vi "skil3.vi"() -> ()   [LabVIEW 2010]
uses:
  <vilib>/Utility/miscctls.llb/LVRectTypeDef.ctl
  lib/Global 2.vi
  <vilib>/Platform/browser.llb/Open URL in Default Browser (path).vi
panel:
  in  "Ed":bool
  in  "fv":bool
  in  "tm":bool
  out "mode":bool caption="Расписание"
  out "Table":string[][](table)
  out "User":string
  out "Device:Temperature":dbl format="%#4.0f"
  out "GPS:Status":i32(ring) items=["Uninitialized", "Antenna Error", "No Useable Satellites", "One Useable Satellite", "Two Useable Satellites", "Three Useable Satellites", "No GPS Time", "PDOP Too High", "Unuseable Satellite", "Fix Rejected", "Self Survey Complete", "Self Survey Not Complete"]
  out "d_h_m_s":dbl caption="в работе (дни, часы, минуты, секунды)" format="%<%D:%H:%M:%S>t"
  out "# elements in queue":i32 caption="Импульсов"
  in  "indexhtm":bool
  in  "stop 2":bool
  out "Get":bool caption="Датчики"
  out "Save2disk":bool caption="Диск"
  out "Files":i32 caption="Необработано"
  out "Send":bool caption="Сервер"
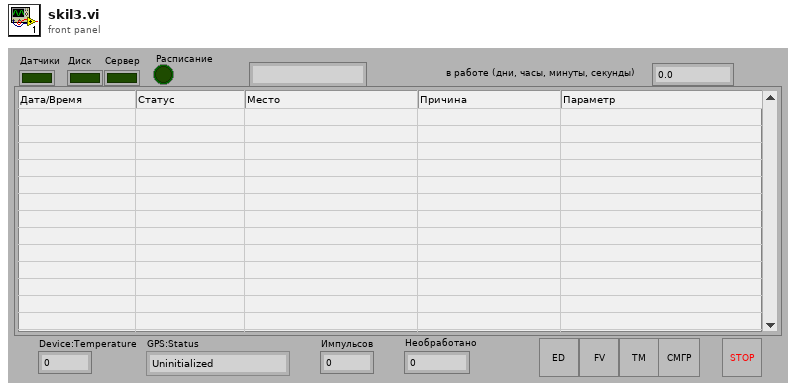
[diagram p1: front panel]
types:
  T1 = cluster{"seconds since 1Jan1904":timestamp, "error out":errorcluster}
  T2 = typedef "LVRectTypeDef.ctl" = cluster{"Left":i16, "Top":i16, "Right":i16, "Bottom":i16}
  T3 = cluster{cluster{"actualSamples":i32, "absoluteInitialX":dbl, "relativeInitialX":dbl, "xIncrement":dbl, "offset":dbl, "gain":dbl, "reserved1":dbl, "reserved2":dbl}[], "wfm":i16[][]}
  T4 = cluster{"adc handle":refnum<k15>, "PN":string, "KR":string}
  T5 = cluster{"seconds since 1Jan1904":timestamp, "error out":errorcluster}[]
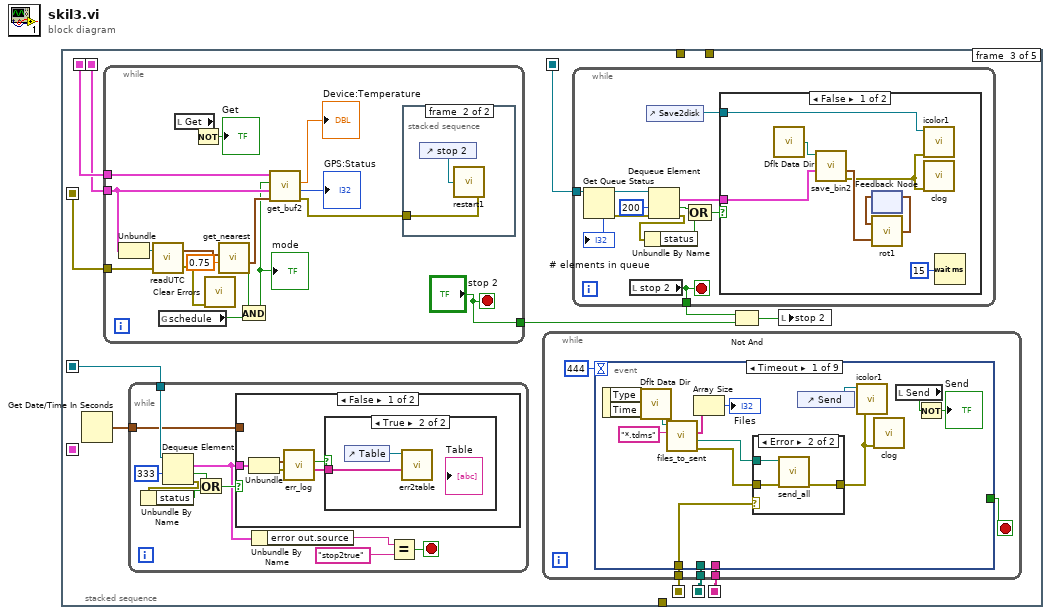
[diagram p0: block diagram]
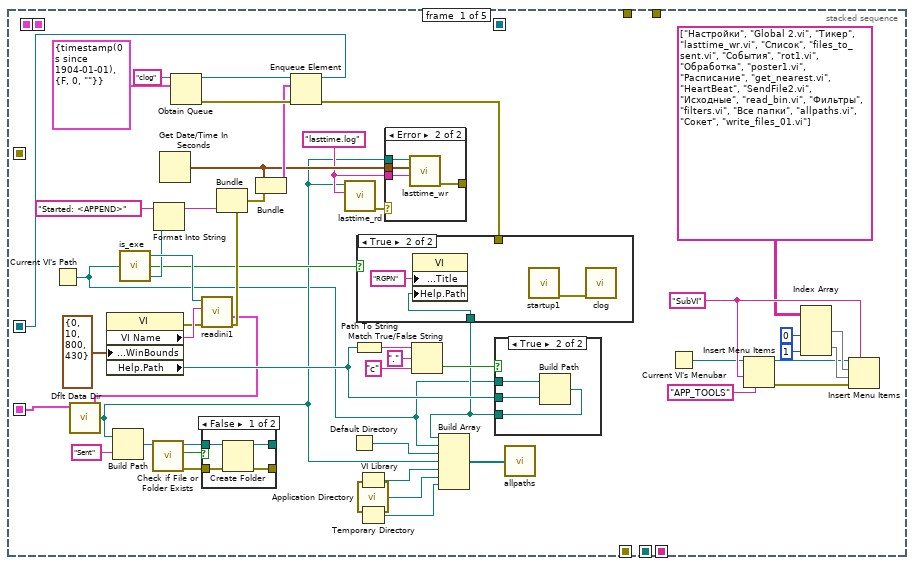
[diagram p2: hidden frame]
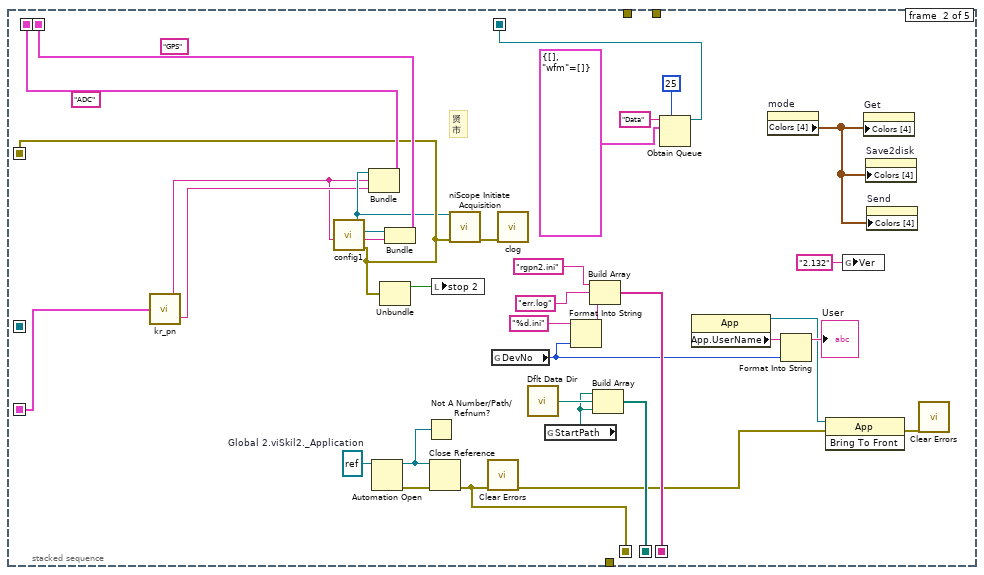
[diagram p7: hidden frame]
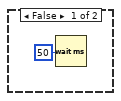
[diagram p8: hidden frame]
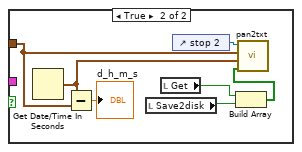
[diagram p9: hidden frame]
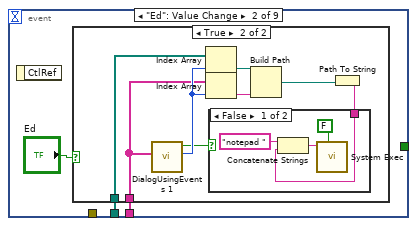
[diagram p11: hidden frame]
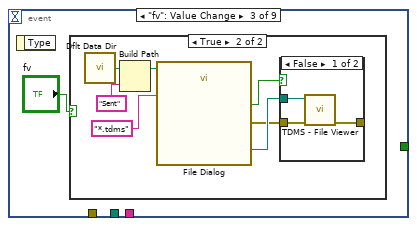
[diagram p14: hidden frame]
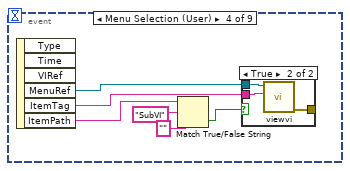
[diagram p17: hidden frame]
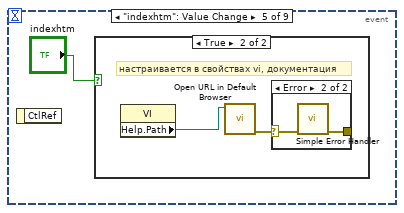
[diagram p19: hidden frame]
diagram:
  n1 = stacked-sequence {
    seq-local: [_ w93 _ _ _] -> [_ _ w113 w269 _]
    seq-local: [_ w101 _ _ _] -> [_ _ w112 w275 _]
    seq-local: [_ w97 _ _ _] -> [_ _ w110 w264 _]
    seq-local: [_ w98 _ _ _] -> [_ _ w111 w266 _]
    seq-local: [w20 _ _ _ _] -> [_ _ w109 w260 _]
    seq-local: [_ w84 _ _ _] -> [_ _ w108 _ _]
    seq-local: [_ w83 _ _ _] -> [_ _ w107 _ _]
    seq-local: [_ w74 _ _ _] -> [_ _ w102 _ _]
    seq-local: [w1 _ _ _ _] -> [_ w69 _ _ _]
    tunnel: [_ _ _ w256 _] -> _
    tunnel: [_ _ _ w255 _] -> _
    tunnel: [_ _ _ w252 _] -> _
    frame #0 {
      w6 = "lasttime.log" ("name or relative path")
      w40 = "SubVI"
      n2 = Current VI's Path() -> (path=w3:path)
      n3 = call <vilib>:"Dflt Data Dir.vi"() -> ("App:Default Data Directory"=w4:path)
      n4 = property class="VI"("Front Panel.WinBounds"=T2 {"Left"=0, "Top"=10, "Right"=800, "Bottom"=430} ("Front Panel Window:Window Bounds")) -> (error out=w47:errorcluster, "VI Name"=w49:string, "Help.Path"=w13:path)  [unwired: 2 in, 1 out]
      n5 = Build Path(base path=w4, name or relative path="Sent") -> (appended path=w44:path)
      n6 = call "is_exe.vi"("path"=w3) -> ("actual path"=w21:path, "exe?"=w19:bool, "ini path"=w48:path)  [unwired: 2 in]
      n7 = call <vilib>:"Check if File or Folder Exists.vi"("path"=w44) -> ("error out"=w41:errorcluster, "file or folder exists?"=w43:bool, "dup path"=w42:path)  [unwired: 8 in]
      n8 = Format Into String(initial string="Started: <APPEND>" ("string"), w21) -> (resulting string=w24:string)  [unwired: 2 in, 1 out]
      n9 = Get Date/Time In Seconds() -> (seconds since 1Jan1904=w7:timestamp)
      n10 = Obtain Queue(name (unnamed)="clog", element data type=T1 {"seconds since 1Jan1904"=timestamp(0 s since 1904-01-01), "error out"={"status"=FALSE, "code"=0, "source"=""}} ("output cluster")) -> (queue out=w28:refnum<queue>, error out=w27:errorcluster)  [unwired: 3 in, 1 out]
      n11 = call "readini1.vi"("error in (no error)"=w47, "section"=w49, "configuration file path"=w48) -> ("error out"=w26:errorcluster, "Dev_Gr"=w1:cluster{"DevNo":i32, "Group":string}[])  [unwired: 1 in, 2 out]
      n12 = case shown="False" w43 {
        tunnel: w42 -> [w64 w66]
        tunnel: w41 -> [w63 w65]
        tunnel: [w62 w66] -> _
        tunnel: [w61 w65] -> _
        frame False {
          n13 = Create Folder(path (use dialog)=w64, error in=w63) -> (created path=w62:path, error out=w61:errorcluster)  [unwired: 1 in, 1 out]
        }
        frame True {
        }
      }
      n14 = Bundle(cluster=w26, "source"=w24) -> (w23:errorcluster)  [unwired: 2 in]
      n15 = Bundle("seconds since 1Jan1904"=w7, "error out"=w23) -> (w22:T1)  [unwired: 1 in]
      n16 = Enqueue Element(queue=w28, element=w22, error in (no error)=w27) -> (queue out=w20:refnum<queue>, error out=w18:errorcluster)  [unwired: 1 in, 1 out]
      n17 = call "lasttime_rd.vi"("name or relative path"=w6, "base path"=w4) -> ("error out"=w5:errorcluster)  [unwired: 3 in, 2 out]
      n18 = Default Directory() -> (w15:path)
      n19 = Path To String(path=w13) -> (string=w12:string)
      n20 = VI Library() -> (path=w16:path)
      n21 = call <vilib>:"Application Directory.vi"() -> ("Application Directory"=w2:path)
      n22 = Temporary Directory() -> (w17:path)
      n23 = case shown="Error" w5 {
        tunnel: w7 -> [_ w53]
        tunnel: w6 -> [_ w52]
        tunnel: w4 -> [_ w51]
        tunnel: [_ w50] -> _
        frame No Error {
        }
        frame Error {
          n24 = call "lasttime_wr.vi"("name"=w52, "time stamp"=w53, "start Path"=w51) -> ("error out"=w50:errorcluster)  [unwired: 3 in, 1 out]
        }
      }
      n25 = Match True/False String(2:"c" ("false string"), 3:"." ("true string"), 4:w12) -> (0:w9:bool)  [unwired: 1 out]
      n26 = case shown="True" w9 {
        tunnel: w13 -> [w54 w57]
        tunnel: [w54 w56] -> w8
        tunnel: w3 -> [_ w55]
        frame False {
        }
        frame True {
          n27 = Build Path(base path=w55, name or relative path=w57) -> (appended path=w56:path)
        }
      }
      n28 = case shown="True" w19 {
        tunnel: w18 -> [_ _]
        tunnel: w8 -> [_ w58]
        frame False {
        }
        frame True {
          n29 = property class="VI"("Front Panel.Title"="RGPN" ("Front Panel Window:Title"), "Help.Path"=w58) -> ()  [unwired: 2 in, 2 out]
          n30 = call "startup1.vi"() -> ("error out"=w59:errorcluster)  [unwired: 7 in]
          n31 = call "clog.vi"("error"=w59) -> ()  [unwired: 7 in]
        }
      }
      n32 = Build Array(w8, w3, w15, w4, w16, w2, w17) -> (w14:path[])
      n33 = call "allpaths.vi"("Array"=w14) -> ()
      n34 = Current VI's Menubar() -> (w31:refnum<k9>)
      n35 = Insert Menu Items(4:"APP_TOOLS" ("after item"), 7:w40, 9:w31) -> (0:w33:errorcluster, 3:w32:refnum<k9>)  [unwired: 3 in, 1 out]
      n36 = Index Array(array=string[][] [["Настройки", "Global 2.vi"], ["Тикер", "lasttime_wr.vi"], ["Список", "files_to_sent.vi"], ["События", "rot1.vi"], ["Обработка", "poster1.vi"], ["Расписание", "get_nearest.vi"], ["HeartBeat", "SendFile2.vi"], ["Исходные", "read_bin.vi"], ["Фильтры", "filters.vi"], ["Все папки", "allpaths.vi"], ["Сокет", "write_files_01.vi"]], index (col) #1=0 ("disabled index (col)"), index (col) #2=1 ("index (col)")) -> (element #1=w36:string[], element #2=w37:string[])  [unwired: 2 in]
      n37 = Insert Menu Items(5:w40, 6:w33, 7:w37, 8:w36, 9:w32) -> ()  [unwired: 1 in, 3 out]
    }
    frame #1 {
      w75 = refnum<k7> refnum  # Global 2.viSkil2._Application
      (unwired) "GPS"
      (unwired) "ADC"
      # "贤\n市"
      n38 = call "kr_pn.vi"("Dev_Gr"=w69) -> ("KR"=w68:string, "PN"=w67:string)
      n39 = call "config1.vi"("ChList"=w67) -> ("error out"=w93:errorcluster, "trig"=w99:tag, "gps handle"=w100:refnum<k15>, "adc handle"=w91:refnum<k15>)  [unwired: 3 in]
      n40 = Bundle("adc handle"=w91, "PN"=w67, "KR"=w68) -> (w98:T4)  [unwired: 1 in]
      n41 = Automation Open(Automation Refnum=w75) -> (Automation Refnum=w70:refnum<k7>, error out=w76:errorcluster)  [unwired: 3 in]
      n42 = Unbundle(w93) -> ("status"=w95:bool)  [unwired: 2 out]
      n43 = Bundle("gps handle"=w100, "trig"=w99) -> (w97:cluster{"gps handle":refnum<k15>, "trig":tag})  [unwired: 1 in]
      n44 = Not A Number/Path/Refnum?(number/path/refnum=w70) -> ()  [unwired: 1 out]
      n45 = Close Reference(reference=w70, error in (no error)=w76) -> (error out=w74:errorcluster)
      n46 = local write "stop 2"(w95) -> ()
      n47 = call <instrlib>:"niScope Initiate Acquisition.vi"("instrument handle"=w91, "error in"=w93) -> ("error out"=w92:errorcluster)  [unwired: 12 in, 1 out]
      n48 = call <vilib>:"Clear Errors.vi"("error in (no error)"=w74) -> ("error out"=w73:errorcluster)  [unwired: 6 in]
      n49 = global read "Global 2.vi" "DevNo"() -> (w78:i32)
      n50 = call "clog.vi"("error"=w92) -> ()  [unwired: 7 in]
      n51 = call <vilib>:"Dflt Data Dir.vi"() -> ("App:Default Data Directory"=w87:path)
      n52 = global read "Global 2.vi" "StartPath"() -> (w81:path)
      n53 = Format Into String(format string="%d.ini", w78) -> (resulting string=w85:string)  [unwired: 2 in, 1 out]
      n54 = Build Array("rgpn2.ini" ("element"), "err.log", w85) -> (w83:string[])
      n55 = Build Array(w81, w87, w81) -> (w84:path[])
      n56 = Obtain Queue(max queue size (-1, unlimited)=25, name (unnamed)="Data", element data type=T3 {[], "wfm"=[]} ("Cluster")) -> (queue out=w101:refnum<queue>)  [unwired: 2 in, 2 out]
      n57 = property class="App"() -> (reference out=w72:refnum<vi>, "App.UserName"=w80:string)  [unwired: 2 in, 1 out]
      n58 = property on="mode" class="Bool (strict)"() -> ("Colors [4]"=w94:cluster{u32, u32}[])  [unwired: 2 in, 2 out]
      n59 = Format Into String(initial string=w80, w78) -> (resulting string=→"User":string)  [unwired: 2 in, 1 out]
      n60 = invoke class="App" method="Bring To Front"(reference=w72, error in=w73) -> (error out=w71:errorcluster)  [unwired: 1 in, 2 out]
      n61 = global write "Global 2.vi" "Ver"("2.132" ("Ver")) -> ()
      n62 = property on="Get" class="Bool (strict)"("Colors [4]"=w94) -> ()  [unwired: 2 in, 2 out]
      n63 = property on="Save2disk" class="Bool (strict)"("Colors [4]"=w94) -> ()  [unwired: 2 in, 2 out]
      n64 = property on="Send" class="Bool (strict)"("Colors [4]"=w94) -> ()  [unwired: 2 in, 2 out]
      n65 = call <vilib>:"Clear Errors.vi"("error in (no error)"=w71) -> ()  [unwired: 6 in, 1 out]
    }
    frame #2 {
      n66 = Get Date/Time In Seconds() -> (seconds since 1Jan1904=w106:timestamp)
      n67 = while {
        tunnel: w113 -> [w236]
        tunnel: w110 -> [w246]
        tunnel: w111 -> [w244]
        tunnel: ["stop 2"] -> w104
        stop <- "stop 2" stop-if-true
        n68 = Unbundle(w246) -> ("gps handle"=w245:refnum<k15>)  [unwired: 1 out]
        n69 = call "readUTC.vi"("error out 2"=w236, "gps handle"=w245) -> ("error out"=w231:errorcluster, "time"=w247:timestamp)
        n70 = global read "Global 2.vi" "schedule"() -> (w233:bool)
        n71 = local read "Get"() -> (w240:bool)
        n72 = Not(x=w240) -> (.not. x?=→"Get":bool)
        n73 = call <vilib>:"Clear Errors.vi"("error in (no error)"=w231) -> ()  [unwired: 6 in, 1 out]
        n74 = call "get_nearest.vi"("interval_sec"=0.75, "current time"=w247) -> ("found"=w235:bool, "next_TimeStamp"=w242:timestamp)  [unwired: 3 in, 1 out]
        n75 = And(x=w235, y=w233) -> (x .and. y?=w234:bool)
        "mode" <- w234
        n76 = call "get_buf2.vi"("time GPS"=w242, "Sync cluster"=w246, "Boolean"=w234, "Scope Cluster"=w244) -> ("error out"=w239:errorcluster, "Timing:GPS:Status"=→"GPS:Status":i32, "Device:Temperature"=→"Device:Temperature":dbl)  [unwired: 1 in]
        n77 = stacked-sequence {
          tunnel: w239 -> [w248 w251]
          frame #0 {
            n78 = control-ref of="Get"() -> (w249:refnum<vi>)
            n79 = call "clog.vi"("error"=w248) -> ()  [unwired: 7 in]
            n80 = call "icolor1.vi"("error in (no error)"=w248, "Bool Refnum"=w249) -> ()  [unwired: 6 in]
          }
          frame #1 {
            n81 = control-ref of="stop 2"() -> (w250:refnum<vi>)
            n82 = call "restart1.vi"("error in"=w251, "Bool Refnum"=w250) -> ()
          }
        }
      }
      n83 = while {
        tunnel: w109 -> [w123]
        tunnel: w106 -> [w118]
        stop <- w116 stop-if-true
        n84 = Dequeue Element(queue=w123, timeout in ms (-1)=333) -> (element=w115:T1, timed out?=w120:bool, error out=w122:errorcluster)  [unwired: 1 in, 1 out]
        n85 = Unbundle By Name(w122) -> ("status"=w121:bool)
        n86 = Or(x=w120, y=w121) -> (x .or. y?=w119:bool)
        n87 = case shown="False" w119 {
          tunnel: w115 -> [w129 _]
          tunnel: w118 -> [_ w137]
          frame False {
            n88 = Unbundle(w129) -> ("seconds since 1Jan1904"=w128:timestamp, "error out"=w127:errorcluster)
            n89 = call "err_log.vi"("error In"=w127, "time stamp"=w128) -> ("err_table"=w126:string[], "do?"=w125:bool)  [unwired: 4 in]
            n90 = case shown="True" w125 {
              tunnel: w126 -> [_ w132]
              frame False {
                n91 = Wait (ms)(milliseconds to wait=u32 50) -> ()  [unwired: 1 out]
              }
              frame True {
                n92 = control-ref of="Table"() -> (w131:refnum<vi>)
                n93 = call "err2table.vi"("err_table"=w132, "Tbl Refnum"=w131) -> ()  [unwired: 6 in]
              }
            }
          }
          frame True {
            n94 = Get Date/Time In Seconds() -> (seconds since 1Jan1904=w138:timestamp)
            n95 = Subtract(x=w138, y=w137) -> (x-y=→"d_h_m_s":dbl)
            n96 = local read "Save2disk"() -> (w134:bool)
            n97 = local read "Get"() -> (w135:bool)
            n98 = control-ref of="stop 2"() -> (w136:refnum<vi>)
            n99 = Build Array(w135, w134) -> (w133:bool[])
            n100 = call "pan2txt.vi"("Boolean array"=w133, "seconds since 1Jan1904"=w138, "started"=w137, "stop button"=w136) -> ()  [unwired: 4 in]
          }
        }
        n101 = Unbundle By Name(w115) -> ("error out.source"=w114:string)
        n102 = Equal?(x=w114, y="stop2true" ("source")) -> (x = y?=w116:bool)
      }
      n103 = while {
        tunnel: w108 -> [w142]
        tunnel: w107 -> [w141]
        tunnel: w102 -> [w140]
        stop <- w143 stop-if-true
        n104 = event shown="[0] Timeout" {
          selector: _ -> [_ _ _ _ _ _ _ _ _]
          dyn-events: _ -> [_ _ _ _ _ _ _ _ _]
          timeout: 444 -> [_ _ _ _ _ _ _ _ _]
          tunnel: [_ _ _ _ _ _ w205 _ _] -> w143
          tunnel: w142 -> [_ w161 _ _ _ _ _ _ _]
          tunnel: w141 -> [_ w160 _ _ _ _ _ _ _]
          tunnel: w140 -> [w145 _ _ _ _ _ _ _ _]
          event Timeout {
            n105 = event-data() -> ()  [unwired: 1 in, 2 out]
            n106 = call <vilib>:"Dflt Data Dir.vi"() -> ("App:Default Data Directory"=w155:path)
            n107 = call "files_to_sent.vi"("pattern"="*.tdms", "Directory"=w155) -> ("error IO"=w151:errorcluster, "file_1 path"=w146:path, "names"=w152:string[])  [unwired: 2 in, 1 out]
            n108 = Array Size(array=w152) -> (size(s)=→"Files":i32)
            n109 = case shown="Error" w145 {
              tunnel: w151 -> [w156 w159]
              tunnel: [w156 w158] -> w147
              tunnel: w146 -> [_ w157]
              frame No Error {
              }
              frame Error {
                n110 = call "send_all.vi"("error IO"=w159, "file path"=w157) -> ("error out"=w158:errorcluster)  [unwired: 3 in, 2 out]
              }
            }
            n111 = control-ref of="Send"() -> (w148:refnum<vi>)
            n112 = call "icolor1.vi"("error in (no error)"=w147, "Bool Refnum"=w148) -> ()  [unwired: 6 in]
            n113 = call "clog.vi"("error"=w147) -> ()  [unwired: 7 in]
            n114 = local read "Send"() -> (w153:bool)
            n115 = Not(x=w153) -> (.not. x?=→"Send":bool)
          }
          event "Ed": Value Change {
            n116 = event-data() -> ()  [unwired: 1 in, 1 out]
            n117 = case shown="True" "Ed" {
              tunnel: w161 -> [_ w164]
              tunnel: w160 -> [_ w163]
              frame False {
              }
              frame True {
                n118 = call "DialogUsingEvents 1.vi"("Strings []"=w163) -> ("Numeric"=w170:i32, "Cancelled?"=w165:bool)  [unwired: 8 in, 1 out]
                n119 = Index Array(array=w164, index=w170) -> (element=w169:path)
                n120 = Index Array(array=w163, index=w170) -> (element=w168:string)
                n121 = Build Path(base path=w169, name or relative path=w168) -> (appended path=w167:path)
                n122 = Path To String(path=w167) -> (string=w166:string)
                n123 = case shown="False" w165 {
                  tunnel: w166 -> [w173 _]
                  frame False {
                    n124 = Concatenate Strings("notepad " ("string"), w173) -> (w172:string)
                    n125 = call <vilib>:"System Exec.vi"("wait until completion? (T)"=FALSE, "command line"=w172) -> ()  [unwired: 6 in, 4 out]
                  }
                  frame True {
                  }
                }
              }
            }
          }
          event "fv": Value Change {
            n126 = event-data() -> ()  [unwired: 1 in, 1 out]
            n127 = case shown="True" "fv" {
              frame False {
              }
              frame True {
                n128 = call <vilib>:"Dflt Data Dir.vi"() -> ("App:Default Data Directory"=w177:path)
                n129 = Build Path(base path=w177, name or relative path="Sent") -> (appended path=w176:path)
                n130 = call "File Dialog"("start path"=w176, "pattern (all files)"="*.tdms") -> ("selected path"=w182:path, "cancelled"=w179:bool, "error out"=w181:errorcluster)  [unwired: 10 in, 1 out]
                n131 = case shown="False" w179 {
                  tunnel: [w185 _] -> _
                  tunnel: w182 -> [w184 _]
                  tunnel: w181 -> [w183 _]
                  frame False {
                    n132 = call <vilib>:"TDMS - File Viewer.vi"("error in (no error)"=w183, "file path"=w184) -> ("error out"=w185:errorcluster)  [unwired: 4 in, 1 out]
                  }
                  frame True {
                  }
                }
              }
            }
          }
          event Menu Selection (User) {
            n133 = event-data() -> ("MenuRef"=w189:refnum<k9>, "ItemTag"=w188:string, "ItemPath"=w187:string)  [unwired: 1 in, 3 out]
            n134 = Match True/False String(2:"" ("false string"), 3:"SubVI" ("true string"), 4:w187) -> (0:w190:bool)  [unwired: 1 out]
            n135 = case shown="True" w190 {
              tunnel: w189 -> [_ w194]
              tunnel: [_ w193] -> _
              tunnel: w188 -> [_ w192]
              frame False {
              }
              frame True {
                n136 = call "viewvi.vi"("item tag"=w192, "menu reference"=w194) -> ("error out"=w193:errorcluster)  [unwired: 5 in]
              }
            }
          }
          event "indexhtm": Value Change {
            n137 = event-data() -> ()  [unwired: 1 in, 1 out]
            n138 = case shown="True" "indexhtm" {
              frame False {
              }
              frame True {
                # "настраивается в свойствах vi, документация"
                n139 = property class="VI"() -> ("Help.Path"=w196:path)  [unwired: 2 in, 2 out]
                n140 = call-poly <vilib>:"Open URL in Default Browser.vi"("path"=w196) -> ("error out"=w197:errorcluster)  [unwired: 5 in, 1 out]
                n141 = case shown="Error" w197 {
                  selector: w197 -> [_ w199]
                  tunnel: [_ w198] -> _
                  frame No Error {
                  }
                  frame Error {
                    n142 = call <vilib>:"Simple Error Handler.vi"("error in (no error)"=w199) -> ("error out"=w198:errorcluster)  [unwired: 4 in, 4 out]
                  }
                }
              }
            }
          }
          event "tm": Value Change {
            n143 = event-data() -> ()  [unwired: 1 in, 1 out]
            n144 = case shown="True" "tm" {
              tunnel: [_ w201] -> _
              frame False {
              }
              frame True {
                n145 = call <vilib>:"System Exec.vi"("run minimized? (F)"=FALSE, "wait until completion? (T)"=FALSE, "command line"="taskmgr") -> ("error out"=w201:errorcluster)  [unwired: 5 in, 3 out]
              }
            }
          }
          event "stop 2": Value Change {
            n146 = event-data() -> ("NewVal"=w205:bool)  [unwired: 1 in, 4 out]
            n147 = case shown="True" w205 {
              frame False {
              }
              frame True {
                n148 = call "clog.vi"("error"=errorcluster {"status"=TRUE, "code"=0, "source"="stop2true"}) -> ()  [unwired: 7 in]
              }
            }
          }
          event Application Instance Close? {
            w207 = TRUE ("Value (Signaling)")
            n149 = event-data() -> ()  [unwired: 1 in, 4 out]
            n150 = property on="stop 2" class="Bool (strict)"("Val(Sgnl)"=w207) -> ()  [unwired: 2 in, 2 out]
            n151 = event-data("Discard?"=w207) -> ()  [unwired: 2 in, 1 out]
          }
          event Panel Close? {
            w208 = TRUE ("Value (Signaling)")
            n152 = event-data() -> ()  [unwired: 1 in, 3 out]
            n153 = property on="stop 2" class="Bool (strict)"("Val(Sgnl)"=w208) -> ()  [unwired: 2 in, 2 out]
            n154 = event-data("Discard?"=w208) -> ()  [unwired: 1 in, 1 out]
          }
        }
      }
      n155 = while {
        tunnel: w112 -> [w219]
        tunnel: [w209] -> w105
        stop <- w209 stop-if-true
        n156 = Get Queue Status(queue=w219) -> (queue out=w218:refnum<queue>, error out=w217:errorcluster, # elements in queue=→"# elements in queue":i32)  [unwired: 2 in, 5 out]
        n157 = local read "stop 2"() -> (w209:bool)
        n158 = control-ref of="Save2disk"() -> (w216:refnum<vi>)
        n159 = Dequeue Element(queue=w218, timeout in ms (-1)=200, error in (no error)=w217) -> (element=w210:T3, timed out?=w213:bool, error out=w214:errorcluster)  [unwired: 1 out]
        n160 = Unbundle By Name(w214) -> ("status"=w212:bool)
        n161 = Compound Arithmetic op=OR(w213, w212) -> (w211:bool)
        n162 = case shown="False" w211 {
          tunnel: w210 -> [w224 _]
          tunnel: w216 -> [w228 _]
          frame False {
            n163 = call <vilib>:"Dflt Data Dir.vi"() -> ("App:Default Data Directory"=w222:path)
            n164 = call "save_bin2.vi"("xz"=w224, "start path"=w222) -> ("error out"=w221:errorcluster, "timestamp"=w223:timestamp)  [unwired: 3 in, 1 out]
            n165 = feedback #1() -> (w225:timestamp[])  [unwired: 1 in]
            n166 = call "rot1.vi"("t0"=w223, "input"=w225) -> ("output array"=w226:timestamp[])
            n167 = feedback-in #1(w226) -> ()
            n168 = call "icolor1.vi"("error in (no error)"=w221, "Bool Refnum"=w228) -> ()  [unwired: 6 in]
            n169 = call "clog.vi"("error"=w221) -> ()  [unwired: 7 in]
            n170 = Wait (ms)(milliseconds to wait=u32 15) -> ()  [unwired: 1 out]
          }
          frame True {
            n171 = local read "Save2disk"() -> (w229:bool)
            n172 = Not(x=w229) -> (.not. x?=→"Save2disk":bool)
          }
        }
      }
      n173 = Not And(1:w104, 2:w105) -> (0:w103:bool)
      n174 = local write "stop 2"(w103) -> ()
    }
    frame #3 {
      n175 = Unbundle(w266) -> ("adc handle"=w265:refnum<k15>)  [unwired: 2 out]
      n176 = call <instrlib>:"niScope Abort.vi"("instrument handle"=w265, "error in"=w269) -> ("instrument handle out"=w277:refnum<k15>, "error out"=w276:errorcluster)  [unwired: 12 in]
      n177 = call <instrlib>:"niScope Close.vi"("instrument handle"=w277, "error in"=w276) -> ("error out"=w270:errorcluster)  [unwired: 13 in]
      n178 = Get Queue Status(queue=w260, return elements? (F)=TRUE) -> (queue out=w258:refnum<queue>, error out=w253:errorcluster, elements=w257:T5)  [unwired: 1 in, 5 out]
      n179 = for {
        tunnel: w257 -> [w280] mode=indexing
        n180 = Unbundle(w280) -> ("seconds since 1Jan1904"=w279:timestamp, "error out"=w278:errorcluster)
        n181 = call "err_log.vi"("error In"=w278, "time stamp"=w279) -> ()  [unwired: 4 in, 2 out]
      }
      n182 = Unbundle(w264) -> ("gps handle"=w263:refnum<k15>, "trig"=w262:tag)
      n183 = call <instrlib>:"niSync Disable Time Stamp Trigger.vi"("error in (no error)"=w270, "terminal"=w262, "instrument handle"=w263) -> ("error out"=w273:errorcluster, "instrument handle out"=w274:refnum<k15>)  [unwired: 6 in]
      n184 = call <instrlib>:"niSync Disconnect Trigger Terminals.vi"("error in (no error)"=w273, "destination terminal"="AllConnected", "source terminal"="AllConnected", "instrument handle"=w274) -> ("error out"=w272:errorcluster, "instrument handle out"=w271:refnum<k15>)  [unwired: 6 in]
      n185 = Release Queue(queue=w258, force destroy? (F)=TRUE, error in (no error)=w253) -> (error out=w252:errorcluster)  [unwired: 2 out]
      n186 = Release Queue(queue=w275, force destroy? (F)=TRUE) -> (error out=w255:errorcluster)  [unwired: 1 in, 2 out]
      n187 = call <instrlib>:"niSync Close.vi"("error in (no error)"=w272, "instrument handle"=w271) -> ("error out"=w256:errorcluster)  [unwired: 9 in]
    }
    frame #4 {
      n188 = Current VI's Path() -> (path=w283:path)
      n189 = call "is_exe.vi"("path"=w283) -> ("exe?"=w282:bool)  [unwired: 2 in, 2 out]
      n190 = Not(x=w282) -> (.not. x?=w281:bool)
      n191 = Quit LabVIEW(quit? (T)=w282) -> ()
      n192 = Request Deallocation(w281) -> ()
    }
  }
